vi "Event Nested Status.vi"(11 "Base Queue jettl in":refnum<class "Base Queue jettl.lvclass">) -> (0 "Event Nested Count":i32, 1 "Event Nested Aliases":string[](array[string]), 2 "Any Exist?":bool)   [LabVIEW 2021, in "jettl.lvlib" / "Base Queue jettl.lvlib" / "Base Queue jettl.lvclass"]
uses:
  Base Queue jettl.lvclass
  Base Queue jettl.lvclass/Base Queue jettl.ctl
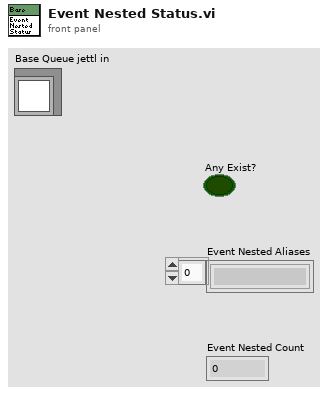
[diagram p1: front panel]
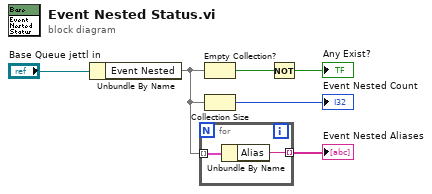
[diagram p0: block diagram]
diagram:
  n1 = Unbundle By Name("Base Queue jettl in") -> ("Event Nested"=w6:map{string, refnum<data-value>})
  n2 = for {
    tunnel: [w7] -> w1 mode=indexing
    tunnel: w6 -> [w8] mode=indexing
    n3 = Unbundle By Name(w8) -> ("Alias"=w7:string)
  }
  "Event Nested Aliases" <- w1
  n4 = Empty Collection?(1:w6) -> (0:w5:bool)
  n5 = Collection Size(1:w6) -> (0:→"Event Nested Count":i32)
  n6 = Not(x=w5) -> (.not. x?=→"Any Exist?":bool)
